vi "AlliGator Compute Smoothed Complex Phasor Array.vi"(8 "error in (no error)":errorcluster, 9 "Time-Gated Reference Decay":cluster{"t Array":dbl[], "I Array":dbl[]}, 10 "Image Array":T17[](array[typedef]), 11 "Sum Image":T17) -> (0 "error out":errorcluster, 1 "Phasor Plot Parameters":T1={"Phasor Frequency"=0.0, "Decay Preprocessing Options & Parameters"={"Background Subtraction Parameters"={"Background Definition Range"={"Min Gate"=0.0, "Max Gate"=0.0}, "Baseline Subtraction Method"=enum."Mean", "Background Subtraction?"=FALSE, "Background File"=path "", "Background Constant"=0.0, "Background Scaling Factor"=1.0, "Background Pile-up Correction"=FALSE, "Background Pixel Well Capacity"=1}, "Decay Preprocessing Parameters"={"Background Subtraction"=FALSE, "Straighten Decay"=FALSE, "Reverse Gates"=FALSE, "1-Normalized Decay"=FALSE, "Smoothen Decay"=FALSE, "Smoothing Parameter"=0.0, "Shift Decay"=FALSE, "Decay Shift Parameters"={"Type"=enum."Default", "Shift"=0.0, "Threshold"=0.0, "Rotate"=FALSE}, "Extrapolate Decay"=FALSE, "Additional Points"=0, "Head Fraction"=0.0, "Pixel-Normalize Decay"=FALSE, "Use Periodicity"=FALSE, "Use Cursors"=FALSE, "Tail Fraction"=0.0, "Use Decay Pre-Processing"=TRUE, "Fold Decay"=FALSE, "# Folds"=1, "[0-1]-Normalized Decay"=FALSE}, "Preprocessing Steps Order"=[]}, "FLI Dataset Modified"=FALSE, "Source Image Settings"={"Low Count Pixels Rejection Options"={"Background Low Threshold Factor"=0.0, "Fixed Low Background Threshold"=0.0, "Reject Low Count Pixels"=FALSE, "Low Percentile"=0.0}, "High Count Pixels Rejection Options"={"Background High Threshold Factor"=0.0, "Fixed High Background Threshold"=20000.0, "Reject High Count Pixels"=FALSE, "High Percentile"=100.0}}, "Data Information"={"Gate Width"=0.0, "Gate Separation"=0.0, "Step (Gate Separation)"=0, "Laser Period"=0.0, "SYNC Period"=0.0, "Channel Name"=0, "Channel Arithmetic"=enum."None", "Pile-up Correction"=FALSE, "Pixel Well Capacity"=1, "Dataset Scaling Factor"=1.0}, "Phasor Plot"={"Phasor Plot Smoothing Options"={"Use Phasor Plot Smoothing"=FALSE, "Kernel Type"=enum."Uniform", "Bin"=1, "Algorithm"=enum."Rapid"}, "Phasor Plot Size"={"H"=0, "V"=0, "Margin"=0.0}, "Selected Image ROI(s)"=FALSE, "All Image ROIs"=FALSE, "Selected Source Image ROI"=0, "Source Image ROIs"=[]}} {"Phasor Plot"."Source Image ROIs"."ROI Descriptor"."Contours"."Type" items=["No Selection", "Point", "Line", "Rectangle", "Oval", "Polygon", "Freehand Region", "Annulus", "Unused2", "Unused3", "Broken Line", "Freehand Line", "Rotated Rectangle"]; "Phasor Plot"."Phasor Plot Smoothing Options"."Bin" min=1 step=2; "Data Information"."Dataset Scaling Factor" min=0.0; "Data Information"."Pixel Well Capacity" min=1 step=1; "Data Information"."Channel Name" items=["Gate"]; "Source Image Settings"."High Count Pixels Rejection Options"."High Percentile" min=0.0 max=100.0; "Source Image Settings"."Low Count Pixels Rejection Options"."Low Percentile" min=0.0 max=100.0; "Decay Preprocessing Options & Parameters"."Decay Preprocessing Parameters"."# Folds" min=1; "Decay Preprocessing Options & Parameters"."Background Subtraction Parameters"."Background Pixel Well Capacity" min=1 step=1}, 2 "Corrected Complex Phasor Array out (VxH)":csg[][](array[numeric]), 3 "Valid Pixel?":bool[][](array[boolean]), 4 "Message":string, 6 "Phasor Array updated":bool)   [LabVIEW 2021, in "AlliGator Phasor Plot.lvlib"]
doc: "Computes the (smoothed) array of single-pixel phasors."
uses:
  AlliGator Phasor Plot.lvlib
  <vilib>/vision/Image Controls.llb/IMAQ Image.ctl
  AlliGator Phasor Plot Parameters v2.ctl
  AlliGator Decay Preprocessing Options.ctl
  AlliGator Background Subtraction Parameters.ctl
  AlliGator Baseline Subtraction Method.ctl
  AlliGator Decay Preprocessing Parameters.ctl
  Graphs/XY Graph/XY Graph Plot Shift Parameters.ctl
  Graphs/XY Graph/XY Graph Plot Shift Method.ctl
  AlliGator Low Count Pixels Rejection Options.ctl
  AlliGator High Count Pixels Rejection Options.ctl
  AlliGator Gate Arithmetic.ctl
  AlliGator Phasor Plot Smoothing Options.ctl
  Arrays/Kernel Type.ctl
  Arrays/Smoothing Algorithm.ctl
  AlliGator Phasor Plot Size.ctl
  Image/Named ROI Description.ctl
  AlliGator Variables List.ctl
  AlliGator Pixel Counts Constraints.ctl
  Phasor/Phasor.lvlib
  AlliGator Decay Processing.lvlib
  AlliGator Globals, Variables & Constants.lvlib
  AlliGator Settings.lvlib
  AlliGator Decay Preprocessing.lvlib
  Graphs/XY Graph/XY Graph Add-Ons.lvlib
  Arrays/Arrays.lvlib
  Image/Image.lvlib
panel:
  # "see the AlliGator License on the block diagram (Ctrl+E or Window:Show Block Diagram)"
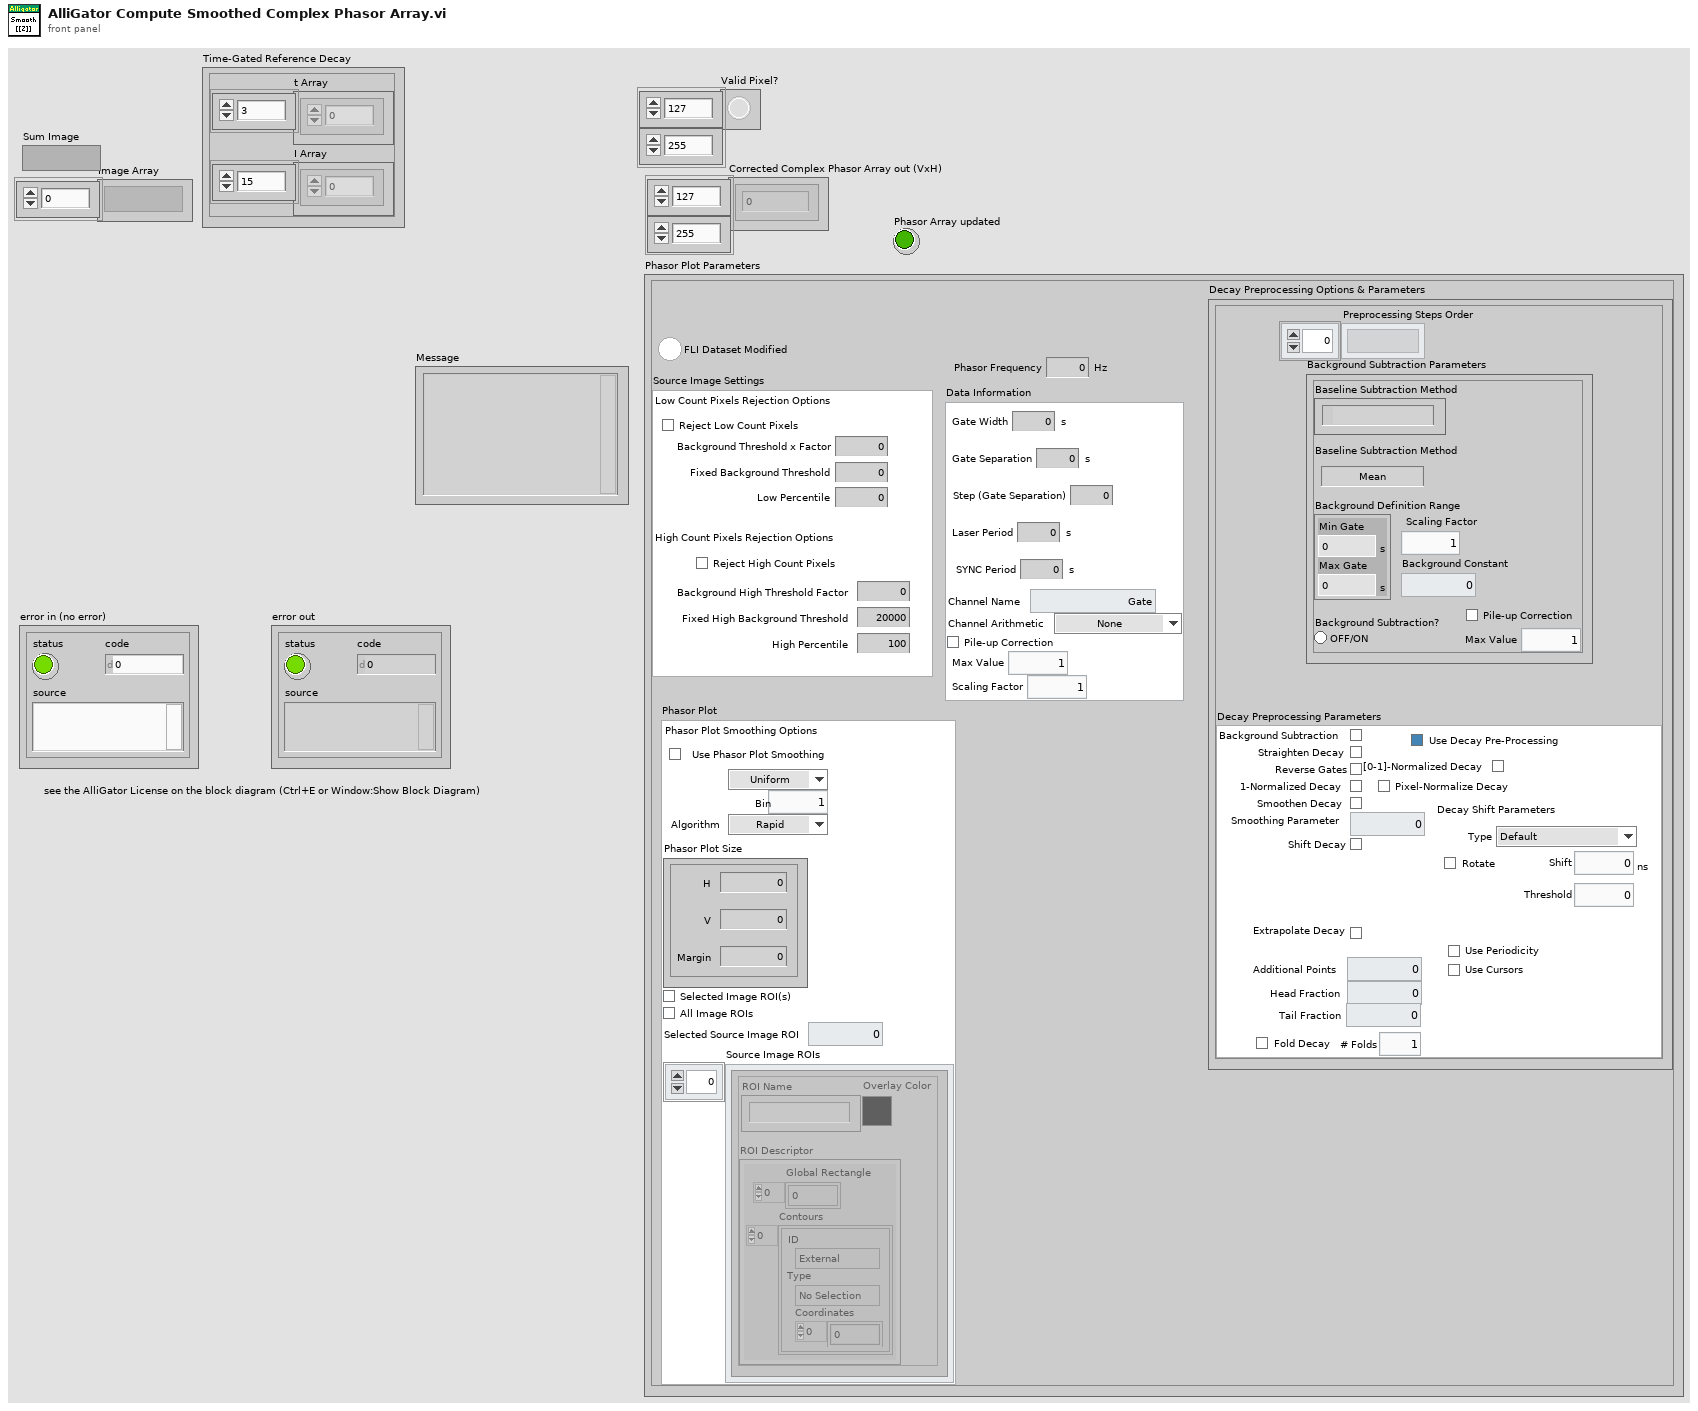
[diagram p1: front panel]
types:
  T1 = typedef "AlliGator Phasor Plot.lvlib/AlliGator Phasor Plot Parameters v2.ctl" = cluster{"Phasor Frequency":dbl[unit], "Decay Preprocessing Options & Parameters":T2, "FLI Dataset Modified":bool, "Source Image Settings":cluster{"Low Count Pixels Rejection Options":T8, "High Count Pixels Rejection Options":T9}, "Data Information":cluster{"Gate Width":dbl[unit], "Gate Separation":dbl[unit], "Step (Gate Separation)":i32, "Laser Period":dbl[unit], "SYNC Period":dbl[unit], "Channel Name":u16, "Channel Arithmetic":T10, "Pile-up Correction":bool, "Pixel Well Capacity":u32, "Dataset Scaling Factor":dbl}, "Phasor Plot":cluster{"Phasor Plot Smoothing Options":T11, "Phasor Plot Size":T14, "Selected Image ROI(s)":bool, "All Image ROIs":bool, "Selected Source Image ROI":i32, "Source Image ROIs":T15[]}}
  T2 = typedef "AlliGator Decay Analysis.lvlib/AlliGator Decay Preprocessing.lvlib/AlliGator Decay Preprocessing Options.ctl" = cluster{"Background Subtraction Parameters":T3, "Decay Preprocessing Parameters":T5, "Preprocessing Steps Order":string[]}
  T3 = typedef "AlliGator Decay Analysis.lvlib/AlliGator Decay Preprocessing.lvlib/AlliGator Background Subtraction Parameters.ctl" = cluster{"Background Definition Range":cluster{"Min Gate":dbl[unit], "Max Gate":dbl[unit]}, "Baseline Subtraction Method":T4, "Background Subtraction?":bool, "Background File":path, "Background Constant":dbl, "Background Scaling Factor":dbl, "Background Pile-up Correction":bool, "Background Pixel Well Capacity":u32}
  T4 = typedef "AlliGator Decay Analysis.lvlib/AlliGator Decay Preprocessing.lvlib/AlliGator Baseline Subtraction Method.ctl" = enum16{"Mean", "Min", "Square Gated Single-Exponential", "File", "Constant"}
  T5 = typedef "AlliGator Decay Analysis.lvlib/AlliGator Decay Preprocessing.lvlib/AlliGator Decay Preprocessing Parameters.ctl" = cluster{"Background Subtraction":bool, "Straighten Decay":bool, "Reverse Gates":bool, "1-Normalized Decay":bool, "Smoothen Decay":bool, "Smoothing Parameter":dbl, "Shift Decay":bool, "Decay Shift Parameters":T6, "Extrapolate Decay":bool, "Additional Points":u32, "Head Fraction":dbl, "Pixel-Normalize Decay":bool, "Use Periodicity":bool, "Use Cursors":bool, "Tail Fraction":dbl, "Use Decay Pre-Processing":bool, "Fold Decay":bool, "# Folds":u32, "[0-1]-Normalized Decay":bool}
  T6 = typedef "XY Graph Add-Ons.lvlib/XY Graph Plot Shift Parameters.ctl" = cluster{"Type":T7, "Shift":dbl[unit], "Threshold":dbl, "Rotate":bool}
  T7 = typedef "XY Graph Add-Ons.lvlib/XY Graph Plot Shift Method.ctl" = enum16{"Default", "CFD", "Threshold", "Cross-Correlation"}
  T8 = typedef "AlliGator Settings.lvlib/AlliGator Low Count Pixels Rejection Options.ctl" = cluster{"Background Low Threshold Factor":dbl, "Fixed Low Background Threshold":dbl, "Reject Low Count Pixels":bool, "Low Percentile":dbl}
  T9 = typedef "AlliGator Settings.lvlib/AlliGator High Count Pixels Rejection Options.ctl" = cluster{"Background High Threshold Factor":dbl, "Fixed High Background Threshold":dbl, "Reject High Count Pixels":bool, "High Percentile":dbl}
  T10 = typedef "AlliGator Settings.lvlib/AlliGator Gate Arithmetic.ctl" = enum16{"None", "INT-G2", "G2/INT*<INT>", "(1 - G2/INT)*<INT>"}
  T11 = typedef "AlliGator Phasor Plot.lvlib/AlliGator Phasor Plot Smoothing Options.ctl" = cluster{"Use Phasor Plot Smoothing":bool, "Kernel Type":T12, "Bin":i32, "Algorithm":T13}
  T12 = typedef "Arrays.lvlib/Kernel Type.ctl" = enum16{"Uniform", "Bilinear", "Gaussian"}
  T13 = typedef "Arrays.lvlib/Smoothing Algorithm.ctl" = enum16{"Rapid", "Thorough"}
  T14 = typedef "AlliGator Phasor Plot.lvlib/AlliGator Phasor Plot Size.ctl" = cluster{"H":i32, "V":i32, "Margin":dbl}
  T15 = typedef "Image.lvlib/Named ROI Description.ctl" = cluster{"ROI Descriptor":T16, "ROI Name":string, "Overlay Color":u32}
  T16 = typedef "ROI Descriptor" = cluster{"Global Rectangle":i32[], "Contours":cluster{"ID":enum32{"External", "Internal"}, "Type":u32, "Coordinates":i32[]}[]}
  T17 = typedef "IMAQ Image.ctl" = refnum<image>
  T18 = typedef "AlliGator Globals, Variables & Constants.lvlib/AlliGator Variables List.ctl" = enum16{"---- GUI ----", "Initialization Status", "State Indicators Refnum", "Original AlliGator Menu Items", "Current Action Loop State", "Script in progress", "Playback", "Loop Playback", "Search ROI Used", "Search ROI", "Decay Graph Max Legend Size", "Intensity Graph Max Legend Size", "Decay Statistics Graph Max Legend Size", "Phasor Graph Max Legend Size", "Phasor Ratio Graph Max Legend Size", "Lifetime Graph Max Legend Size", "---- Files ----", "Export Dataset Frames as Individual Files", "Show Batch Export Help Balloons", "Frames in Dataset", "ptu File Frame Start Indices", "Current Frame in Dataset", "Current Frame Timestamp", "------ Python Plugins ------", "Python Plugins Information", "Python Session", "Valid Python Session?", "---- Source Image ----", "Dataset Loaded", "Dataset Metadata", "Dataset Channel", "Dataset Data Description", "Background Dataset Metadata", "Background Dataset Channel", "Background Dataset Data Description", "Background File Subtraction", "Background File Path", "Background File Pile-up Correction", "Background File Pixel Well Capacity", "Background File Scaling Factor", "Source Image ROIs", "Current Source Image ROI", "Source Image ROI Event Refnum", "X_Source Image Display Range", "X_Source Image Palette Information", "Source Image Palette List", "Source Image Scale", "Current Dataset Load Settings", "Source Image:ROI Overlay Color", "---- Image Profile Window ----", "Image Profile:Overlay ROI in Source Image", "Image Profile Window Event Refnum", "Image Profile:IntensityType", "Image Profile:Intensity Average Type", "Image Profile:Intensity-weighted SDV", "Image Profile:Box Profile Type", "Image Profile Window Open", "Image Profile:Plotted Fit Parameter", "X_Type of Displayed Image", "X_Time Gate Slider", "Dataset Path", "Source Image Overlay to Erase", "Is Displayed Image Accumulated", "White Light Image Modified", "Mask Image Modified", "Macrotime Gate Separation", "------ Phasor Graph -------", "Phasor Graph:Show Line", "---- Phasor Plot ---", "Phasor Plot Parameters Changed", "FLI Dataset Modified since last Phasor Plot Calculation", "Phasor Harmonics Data", "Selected Phasor Harmonics", "Phasor Harmonic Manager Event Refnum", "Phasor Plot ROIs", "Current Phasor Plot ROI", "Phasor Plot ROI Event Refnum", "Phasor Plot Image Reference Points", "Phasor Plot Computed", "Phasor Plot Palette Information", "Phasor Plot Palette List", "Phasor Ratio Palette Information", "Phasor Ratio Palette List", "Phasor Image Scale", "Phasor Plot Image Overlay to Erase", "Phasor Plot Image Elements to Update", "Current Phasor Plot Calculation Parameters", "Current Phasor Calibration Options", "Reset Cumulated Phasor Plot", "Phasor Ratio Reference 1", "Phasor Ratio Lifetime Reference 1", "Phasor Ratio Reference 1 Frequency", "Phasor Ratio Reference 2", "Phasor Ratio Lifetime Reference 2", "Phasor Ratio Reference 2 Frequency", "---- Decay Analysis ----", "Number of Selected Decays to Fit", "LS Fit Results", "LAR Fit Results", "BS Fit Results", "Last Decay Max - Min", "Best Fit Parameters", "Best Fit Parameter Names", "Actual Size X", "Actual Size Y", "Binning X", "Binning Y", "Actual # Gates", "Dataset Number", "Gates to...", "Gates Skipped", "Gates to keep", "Gate Step", "Gate Separation", "Reversed Gates", "Pile-up Correction", "Pixel Well Capacity", "Background Subtracted", "Background Subtraction Method", "Background Definition Range", "Background File (deprecated)", "Number of Dataset Accumulated", "Array of Accumulated Dataset Paths", "Do Averaged Datasets", "Destination File Path", "Process Plot Target", "Use 1/D as Phasor Frequency", "---- Decay Fit Parameter Map -----", "Decay Fit Parameter Map Palette Information", "Decay Fit Parameter Map Palette List", "Local Decay Graph Window Event Refnum", "------- Local Decay Window ---------", "Use normalized IRF for convolution", "----- Miscellaneous ----", "Skippable Dialog Windows Status"}
  T19 = typedef "AlliGator Settings.lvlib/AlliGator Pixel Counts Constraints.ctl" = cluster{"High Count Pixels Rejection Options":T9, "Low Count Pixels Rejection Options":T8}
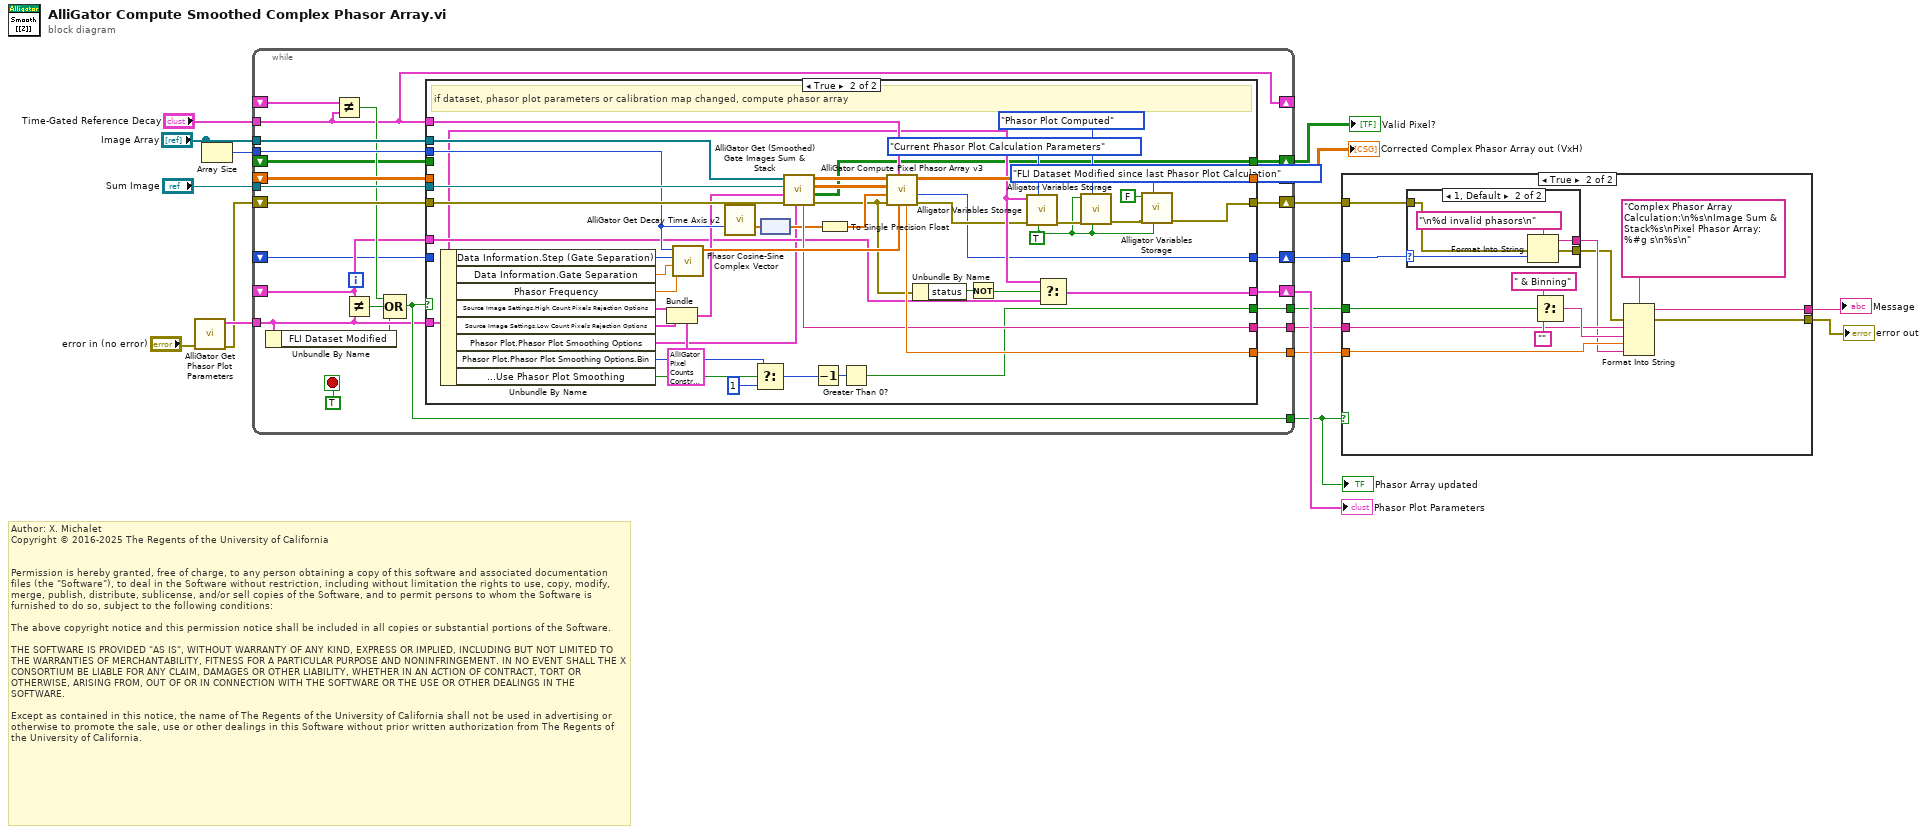
[diagram p0: block diagram]
diagram:
  # "Author: X. Michalet\nCopyright © 2016-2025 The Regents of the University of California\n \n\nPermission is hereby granted, free of charge, to any person obtaining a copy of this software and associated documentation files (the \"Software\"), to deal in the Software without restriction, including without limitation the rights to use, copy, modify, merge, publish, distribute, sublicense, and/or sell copies of the Software, and to permit persons to whom the Software is furnished to do so, subject to the following conditions:\n\nThe above copyright notice and this permission notice shall be included in all copies or substantial portions of the Software.\n\nTHE SOFTWARE IS PROVIDED \"AS IS\", WITHOUT WARRANTY OF ANY KIND, EXPRESS OR IMPLIED, INCLUDING BUT NOT LIMITED TO THE WARRANTIES OF MERCHANTABILITY, FITNESS FOR A PARTICULAR PURPOSE AND NONINFRINGEMENT. IN NO EVENT SHALL THE X CONSORTIUM BE LIABLE FOR ANY CLAIM, DAMAGES OR OTHER LIABILITY, WHETHER IN AN ACTION OF CONTRACT, TORT OR OTHERWISE, ARISING FROM, OUT OF OR IN CONNECTION WITH THE SOFTWARE OR THE USE OR OTHER DEALINGS IN THE SOFTWARE.\n\nExcept as contained in this notice, the name of The Regents of the University of California shall not be used in advertising or otherwise to promote the sale, use or other dealings in this Software without prior written authorization from The Regents of the University of California."
  n1 = call "AlliGator Get Phasor Plot Parameters.vi"("Error In"="error in (no error)") -> ("Error Out"=w11:errorcluster, "Phasor Plot Parameters"=w15:T1)  [unwired: 8 in, 1 out]
  n2 = Array Size(array="Image Array") -> (size(s)=w14:i32)
  n3 = while {
    tunnel: "Image Array" -> [w41]
    tunnel: "Sum Image" -> [w39]
    tunnel: w15 -> [w20]
    tunnel: w14 -> [w38]
    tunnel: [w37] -> w7
    tunnel: [w35] -> w6
    tunnel: [w34] -> w8
    shift-right: [w36] -> w3
    shift-left: w11 -> [w42]
    shift-right: [w29] -> w10
    shift-left: _ -> [w28]
    shift-right: [w40] -> w17
    shift-left: _ -> [w32]
    tunnel: "Time-Gated Reference Decay" -> [w23]
    shift-right: [w23] -> _
    shift-left: _ -> [w31]
    shift-right: [w27] -> w12
    shift-left: _ -> [w26]
    shift-right: [w25] -> w4
    shift-left: _ -> [w24]
    tunnel: [w21] -> w1
    stop <- TRUE stop-if-true
    n4 = Unbundle By Name(w20) -> ("FLI Dataset Modified"=w19:bool)
    n5 = Not Equal?(x=w31, y=w23) -> (x != y?=w30:bool)
    n6 = Not Equal?(x=w28, y=w20) -> (x != y?=w22:bool)
    n7 = Compound Arithmetic op=OR(w30, w22, w19) -> (w21:bool)
    n8 = case shown="True" w21 {
      tunnel: w42 -> [w46 w92]
      tunnel: w41 -> [_ w90]
      tunnel: [w47 w86] -> w40
      tunnel: w39 -> [_ w82]
      tunnel: w38 -> [_ w81]
      tunnel: [_ w77] -> w37
      tunnel: [w46 w51] -> w36
      tunnel: [_ w76] -> w35
      tunnel: [_ w74] -> w34
      tunnel: w20 -> [_ w67]
      tunnel: w32 -> [w47 _]
      tunnel: w23 -> [_ w72]
      tunnel: [w45 w69] -> w29
      tunnel: w28 -> [w45 w68]
      tunnel: [w44 w62] -> w27
      tunnel: w26 -> [w44 _]
      tunnel: [w43 w58] -> w25
      tunnel: w24 -> [w43 _]
      frame False {
        # "If nothing has changed, do not recompute phasor array"
      }
      frame True {
        w50 = TRUE ("Get(F)/Set")
        # "if dataset, phasor plot parameters or calibration map changed, compute phasor array"
        n9 = Unbundle By Name(w67) -> ("Data Information.Step (Gate Separation)"=w91:i32, "Data Information.Gate Separation"=w87:dbl[unit], "Phasor Frequency"=w83:dbl[unit], "Source Image Settings.High Count Pixels Rejection Options"=w80:T9, "Source Image Settings.Low Count Pixels Rejection Options"=w79:T8, "Phasor Plot.Phasor Plot Smoothing Options"=w53:T11, "Phasor Plot.Phasor Plot Smoothing Options.Bin"=w56:i32, "Phasor Plot.Phasor Plot Smoothing Options.Use Phasor Plot Smoothing"=w57:bool)
        n10 = Bundle(cluster=T19 {"High Count Pixels Rejection Options"={"Background High Threshold Factor"=0.0, "Fixed High Background Threshold"=0.0, "Reject High Count Pixels"=FALSE, "High Percentile"=0.0}, "Low Count Pixels Rejection Options"={"Background Low Threshold Factor"=0.0, "Fixed Low Background Threshold"=0.0, "Reject Low Count Pixels"=FALSE, "Low Percentile"=0.0}} ("Pixel Counts Constraints"), "High Count Pixels Rejection Options"=w80, "Low Count Pixels Rejection Options"=w79) -> (w78:T19)
        n11 = call "Phasor Cosine-Sine Complex Vector.vi"("Phasor Frequency"=w83, "Elementary Gate Separation"=w87, "Step"=w91, "# Gates"=w81) -> ("e^j w t_i Vector"=w85:csg[])  [unwired: 7 in]
        n12 = call "AlliGator Get Decay Time Axis v2.vi"("Number of Gates"=w81) -> ("t Array"=w89:dbl[unit][])  [unwired: 14 in]
        n13 = Select(t=w56, s=w57, f=1) -> (s? t:f=w54:i32)
        n14 = node(w89) -> (w73:dbl[])
        n15 = call "AlliGator Get (Smoothed) Gate Images Sum & Stack.vi"("Phasor Plot Smoothing Options"=w53, "Error In"=w92, "Pixel Counts Constraints"=w78, "Sum Image"=w82, "Image Array"=w90) -> ("Error Out"=w60:errorcluster, "[[Valid Pixel]] VxH Array"=w62:bool[][], "Gate Images Stack (N xV xH)"=w88:sgl[][][], "Sum Image (VxH)"=w84:sgl[][], "Message"=w76:string)  [unwired: 2 in]
        n16 = Decrement(x=w54) -> (x-1=w75:i32)
        n17 = To Single Precision Float(number=w73) -> (single precision float=w61:sgl[])
        n18 = Greater Than 0?(x=w75) -> (x > 0?=w74:bool)
        n19 = call "AlliGator Compute Pixel Phasor Array v3.vi"("e^j w t_i Vector"=w85, "Time-Gated Reference Decay"=w72, "Error In"=w60, "t Array"=w61, "Gate Images Stack (NxVxH)"=w88, "Sum Image (V x H)"=w84) -> ("Error Out"=w59:errorcluster, "# Invalid Phasors"=w58:i32, "Pixel Phasors Array (V x H)"=w86:csg[][], "CPU (s)"=w77:dbl)  [unwired: 2 in]
        n20 = Unbundle By Name(w60) -> ("status"=w70:bool)
        n21 = Not(x=w70) -> (.not. x?=w66:bool)
        n22 = call "Alligator Variables Storage.vi"("Get(F)/Set"=w50, "AlliGator Variable"=AlliGator_Variables_List."Current Phasor Plot Calculation Parameters" ("Alligator Variable"), "Error In"=w59, "Data in"=w67) -> ("Error Out"=w65:errorcluster)  [unwired: 5 in, 2 out]
        n23 = Select(t=w67, s=w66, f=w68) -> (s? t:f=w69:T1)
        n24 = call "Alligator Variables Storage.vi"("Get(F)/Set"=w50, "AlliGator Variable"=AlliGator_Variables_List."Phasor Plot Computed" ("Alligator Variable"), "Error In"=w65, "Data in"=w50) -> ("Error Out"=w52:errorcluster)  [unwired: 5 in, 2 out]
        n25 = call "Alligator Variables Storage.vi"("Get(F)/Set"=w50, "AlliGator Variable"=AlliGator_Variables_List."FLI Dataset Modified since last Phasor Plot Calculation" ("Alligator Variable"), "Error In"=w52, "Data in"=FALSE ("Get(F)/Set")) -> ("Error Out"=w51:errorcluster)  [unwired: 5 in, 2 out]
      }
    }
  }
  "Corrected Complex Phasor Array out (VxH)" <- w17
  "Valid Pixel?" <- w12
  "Phasor Plot Parameters" <- w10
  "Phasor Array updated" <- w1
  n26 = case shown="True" w1 {
    tunnel: w8 -> [_ w104]
    tunnel: w7 -> [_ w101]
    tunnel: w6 -> [_ w100]
    tunnel: [_ w99] -> w5
    tunnel: w4 -> [_ w98]
    tunnel: w3 -> [w93 w96]
    tunnel: [w93 w94] -> w2
    frame False {
    }
    frame True {
      n27 = case shown="1, Default" w98 {
        selector: w98 -> [_ w112]
        tunnel: w96 -> [w107 w111]
        tunnel: [w107 w110] -> w95
        tunnel: [_ w108] -> w97
        frame 0 {
        }
        frame 1, Default {
          n28 = Format Into String(format string="\n%d invalid phasors\n", error in=w111, w112) -> (resulting string=w108:string, error out=w110:errorcluster)  [unwired: 1 in]
        }
      }
      n29 = Select(t=" & Binning" ("input 1"), s=w104, f="") -> (s? t:f=w102:string)
      n30 = Format Into String(format string="Complex Phasor Array Calculation:\n%s\nImage Sum & Stack%s\nPixel Phasor Array: %#g s\n%s\n", error in=w95, w100, w102, w101, w97) -> (resulting string=w99:string, error out=w94:errorcluster)  [unwired: 1 in]
    }
  }
  "error out" <- w2
  "Message" <- w5
